vi "Error_Clearing.vi"(8 "error in (no error)":errorcluster) -> (0 "error out":errorcluster)   [LabVIEW 2023]
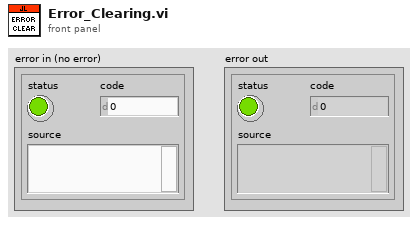
[diagram p1: front panel]
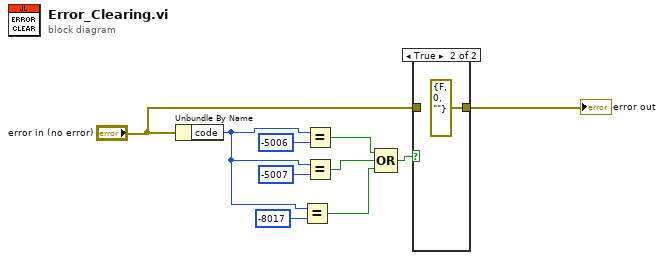
[diagram p0: block diagram]
diagram:
  n1 = Unbundle By Name("error in (no error)") -> ("code"=w3:i32)
  n2 = Equal?(x=w3, y=-8017) -> (x = y?=w1:bool)
  n3 = Equal?(x=w3, y=-5006) -> (x = y?=w8:bool)
  n4 = Equal?(x=w3, y=-5007) -> (x = y?=w7:bool)
  n5 = Compound Arithmetic op=OR(w8, w7, w1) -> (w6:bool)
  n6 = case shown="True" w6 {
    tunnel: [w11 errorcluster {"status"=FALSE, "code"=0, "source"=""} ("error in (no error)")] -> w5
    tunnel: "error in (no error)" -> [w11 _]
    frame False {
    }
    frame True {
    }
  }
  "error out" <- w5
